vi "数字量输出结果.vi"(8 "合格?":bool, 10 "第几个":i32, 11 "第几组":i32) -> ()   [LabVIEW 2010]
uses:
  全局量/自动测试结果.vi
panel:
  # "从0开始"
  # "从0开始"
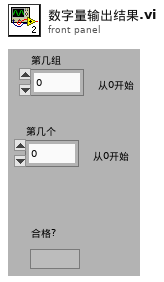
[diagram p1: front panel]
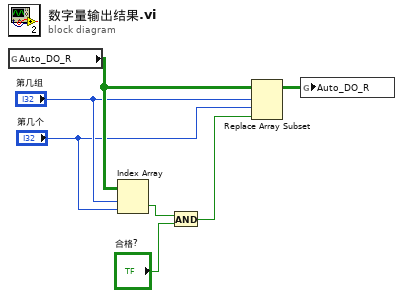
[diagram p0: block diagram]
diagram:
  n1 = global read "自动测试结果.vi" "Auto_DO_R"() -> (w5:bool[][])
  n2 = Index Array(array=w5, index (row)="第几组", index (col)="第几个") -> (element=w7:bool)
  n3 = And(x=w7, y="合格?") -> (x .and. y?=w2:bool)
  n4 = Replace Array Subset(array=w5, new element=w2, index (row)="第几组", index (col)="第几个") -> (w1:bool[][])
  n5 = global write "自动测试结果.vi" "Auto_DO_R"(w1) -> ()
